vi "getDACardSlot.vi"(1 "Card Index":i32) -> (0 "Slot":u16)   [LabVIEW 2011]
uses:
  globals.vi
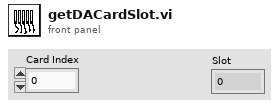
[diagram p1: front panel]
types:
  T1 = cluster{"Relay Card Slots":cluster{"Card 1":u16, "Card 2":u16, "Card 3":u16, "Card 4":u16, "Card 5":u16}, "A/D Card Slots":cluster{"Scanner":u16, "High-Speed A/D":u16, "Timer":u16}, "D/A Cards":cluster{"Quad (10-bit) D/A Card Slots":cluster{"Card 1":u16, "Card 2":u16, "Card 3":u16, "Card 4":u16, "Card 5":u16}, "Single (12-bit) D/A Card Slot":cluster{"Card 6":u16}}}
  T2 = cluster{"Quad (10-bit) D/A Card Slots":cluster{"Card 1":u16, "Card 2":u16, "Card 3":u16, "Card 4":u16, "Card 5":u16}, "Single (12-bit) D/A Card Slot":cluster{"Card 6":u16}}
  T3 = cluster{"Card 1":u16, "Card 2":u16, "Card 3":u16, "Card 4":u16, "Card 5":u16}
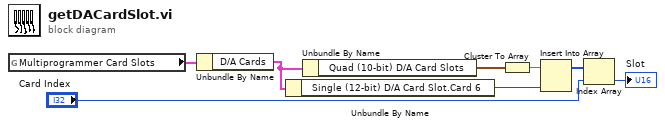
[diagram p0: block diagram]
diagram:
  n1 = global read "globals.vi" "Multiprogrammer Card Slots"() -> (w7:T1)
  n2 = Unbundle By Name(w7) -> ("D/A Cards"=w6:T2)
  n3 = Unbundle By Name(w6) -> ("Single (12-bit) D/A Card Slot.Card 6"=w4:u16)
  n4 = Unbundle By Name(w6) -> ("Quad (10-bit) D/A Card Slots"=w5:T3)
  n5 = Cluster To Array(cluster=w5) -> (array=w2:u16[])
  n6 = Insert Into Array(array=w2, new element=w4) -> (w1:u16[])  [unwired: 1 in]
  n7 = Index Array(array=w1, index="Card Index") -> (element=→"Slot":u16)
